vi "Select XNET Signals.vi"(8 "error in (no error)":errorcluster, 11 "Node Ptr":u64 format="%.0x") -> (0 "error out":errorcluster)   [LabVIEW 2019, in "J1939 Addon System Explorer.lvlib"]
uses:
  J1939 Addon System Explorer.lvlib
  <vilib>/NI VeriStand/Custom Device Tools/Custom Device Utility Library/Search Direction.ctl
  Addon Shared/SubVIs/Constants.vi
  Addon Shared/J1939 Addon Shared.lvlib
  <vilib>/NI VeriStand/Custom Device Tools/Custom Device Utility Library/Custom Device Utility Library.lvlib
panel:
  in  "Tag":string
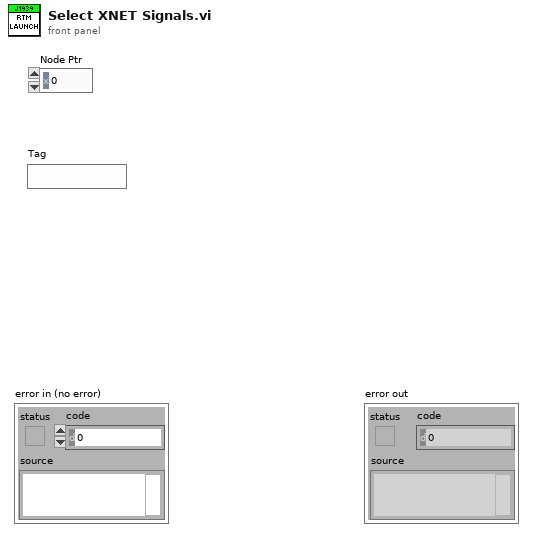
[diagram p1: front panel]
types:
  T1 = typedef "Custom Device Utility Library.lvlib/Search Direction.ctl" = enum16{"Down", "Up"}
  T2 = typedef "Custom Device API.lvlib/Custom Device Item Ref.ctl" = u64
  T3 = typedef "J1939 Addon Shared.lvlib/XNET Settings.ctl" = cluster{"Database":refnum<k21>, "Cluster":refnum<k21>, "Port":string, "Baud rate [Bd]":u32, "Termination":u32, "Incoming Decimation":u32, "Outgoing Decimation":u32}
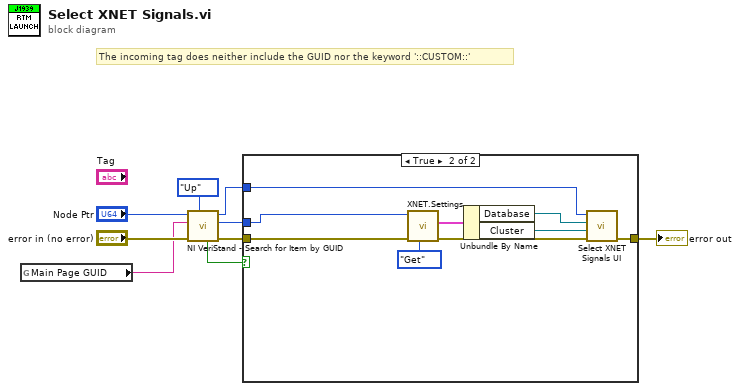
[diagram p0: block diagram]
diagram:
  # "The incoming tag does neither include the GUID nor the keyword '::CUSTOM::'"
  n1 = global read "Constants.vi" "Main Page GUID"() -> (w2:string)
  n2 = call <vilib>:"NI VeriStand - Search for Item by GUID.vi"("Direction (Down)"=Search_Direction."Up", "error in"="error in (no error)", "Item GUID"=w2, "Section Ref in"="Node Ptr") -> ("error out"=w6:errorcluster, "Item Ref"=w5:T2, "Section Ref out"=w3:T2, "Found"=w1:bool)  [unwired: 4 in]
  n3 = case shown="True" w1 {
    tunnel: [w10 w19] -> w9
    tunnel: w6 -> [w10 w12]
    tunnel: w5 -> [_ w13]
    tunnel: w3 -> [_ w17]
    frame False {
    }
    frame True {
      n4 = call "XNET.Settings.vi"("Action"=enum8{"Get", "Set"}."Get", "error in (no error)"=w12, "Parent Ref in"=w13) -> ("error out"=w18:errorcluster, "J1939 XNET Settings"=w14:T3)  [unwired: 6 in, 1 out]
      n5 = Unbundle By Name(w14) -> ("Database"=w16:refnum<k21>, "Cluster"=w15:refnum<k21>)
      n6 = call "Select XNET Signals UI.vi"("error in (no error)"=w18, "XNET Cluster"=w15, "XNET Database"=w16, "Node Ptr"=w17) -> ("error out"=w19:errorcluster)  [unwired: 5 in, 2 out]
    }
  }
  "error out" <- w9
